vi "exercicio_advertencia_temperatura.vi"() -> ()   [LabVIEW 2020]
panel:
  in  "stop":bool
  out "Advertencia":string
  out "Boolean":bool
  in  "Temp max":dbl
  in  "Temp atual":dbl
  in  "Temp min":dbl
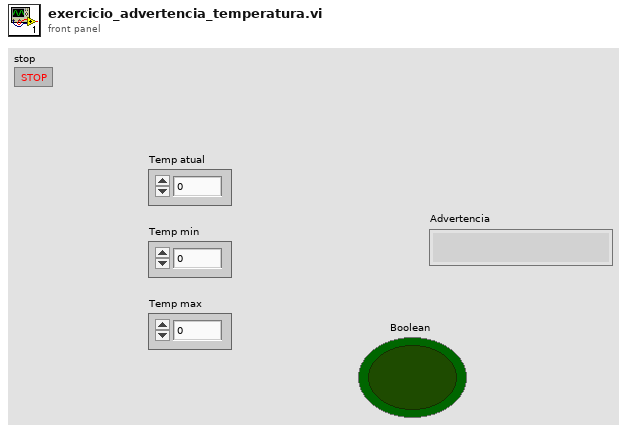
[diagram p1: front panel]
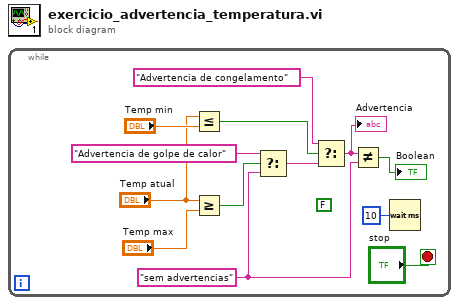
[diagram p0: block diagram]
diagram:
  n1 = while {
    stop <- "stop" stop-if-true
    (unwired) FALSE ("Boolean 2")
    w6 = "sem advertencias"
    n2 = Less Or Equal?(x="Temp atual", y="Temp min") -> (x <= y?=w12:bool)
    n3 = Greater Or Equal?(x="Temp atual", y="Temp max") -> (x >= y?=w10:bool)
    n4 = Select(t="Advertencia de golpe de calor", s=w10, f=w6) -> (s? t:f=w7:string)
    n5 = Select(t="Advertencia de congelamento", s=w12, f=w7) -> (s? t:f=w11:string)
    "Advertencia" <- w11
    n6 = Not Equal?(x=w11, y=w6) -> (x != y?=→"Boolean":bool)
    n7 = Wait (ms)(milliseconds to wait=u32 10) -> ()  [unwired: 1 out]
  }
